vi "sortByChannel.vi"(8 "error in (no error)":errorcluster, 11 "RfOutputData in":refnum<class "RfOutputData.lvclass">) -> (0 "error out":errorcluster, 2 "sortedData":T1(array[cluster]), 3 "RfOutputData out":refnum<class "RfOutputData.lvclass">)   [LabVIEW 2009, in "DataMappers.lvlib" / "RfOutputData.lvclass"]
uses:
  RfOutputData.lvclass
  DatabaseHelpers/Database Objects/Channel/RfOutputChannel/RfOutputChannel.lvclass
  RfOutputData.lvclass/RfOutputData.ctl
  DatabaseHelpers/Database Objects/Channel/Channel.lvclass
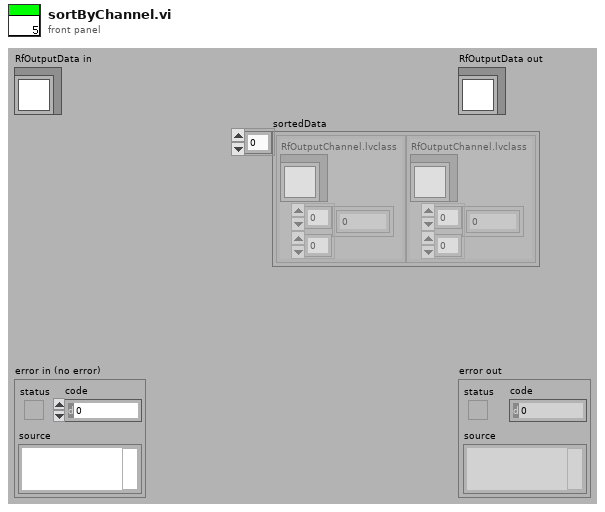
[diagram p1: front panel]
types:
  T1 = cluster{"RfOutputChannel.lvclass":refnum<class "RfOutputChannel.lvclass">, dbl[][]}[]
  T2 = cluster{"rfChannel":refnum<class "RfOutputChannel.lvclass">, "dataValue":dbl, "calibratedFreq":dbl, "calibratedPhase":dbl, "time":dbl}[]
  T3 = cluster{"rfChannel":refnum<class "RfOutputChannel.lvclass">, "dataValue":dbl, "calibratedFreq":dbl, "calibratedPhase":dbl, "time":dbl}
  T4 = cluster{"rfChannel":refnum<class "RfOutputChannel.lvclass">, dbl[][]}
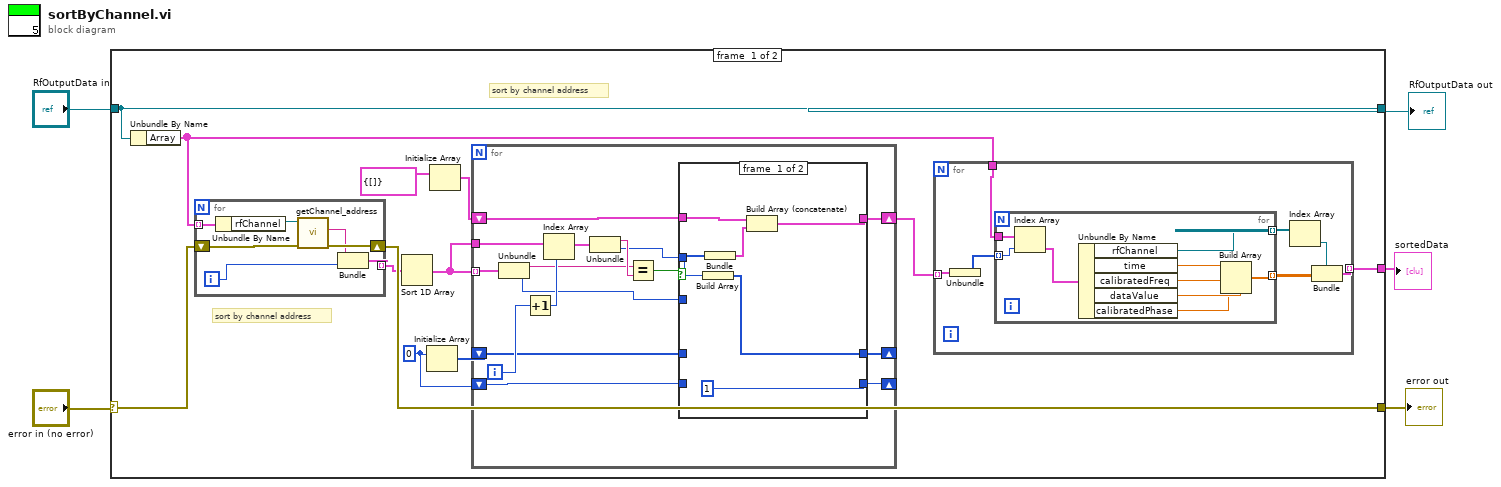
[diagram p0: block diagram]
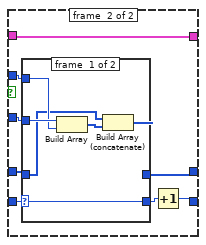
[diagram p2: hidden frame]
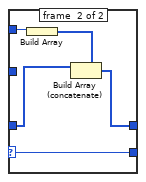
[diagram p3: hidden frame]
diagram:
  n1 = case shown="No Error" "error in (no error)" {
    selector: "error in (no error)" -> [w17 w84]
    tunnel: [w16 w84] -> w4
    tunnel: [w15 w83] -> w2
    tunnel: "RfOutputData in" -> [w15 w83]
    tunnel: [w6 _] -> w1
    frame #0 {
      w9 = 0
      # "sort by channel address"
      # "sort by channel address"
      n2 = Unbundle By Name(w15) -> ("Array"=w7:T2)
      n3 = for {
        tunnel: w7 -> [w82] mode=indexing
        shift-right: [w79] -> w16
        shift-left: w17 -> [w80]
        tunnel: [w77] -> w8 mode=indexing
        i -> [w78]
        n4 = Unbundle By Name(w82) -> ("rfChannel"=w81:refnum<class "RfOutputChannel.lvclass">)
        n5 = call "getChannel_address.vi"("error in (no error)"=w80, "Channel.lvclass in"=w81) -> ("error out"=w79:errorcluster, "channel_address"=w76:string)  [unwired: 7 in, 1 out]
        n6 = Bundle("channel_address"=w76, w78) -> (w77:cluster{"channel_address":string, i32})  [unwired: 1 in]
      }
      n7 = Sort 1D Array(array=w8) -> (sorted array=w14:cluster{"channel_address":string, i32}[])
      n8 = Initialize Array(w9) -> (w13:i32[])  [unwired: 1 in]
      n9 = Initialize Array(cluster{i32[]} {[]} ("output cluster")) -> (w11:cluster{i32[]}[])  [unwired: 1 in]
      n10 = for {
        tunnel: w14 -> [w49] mode=indexing
        tunnel: w14 -> [w48]
        shift-right: [w39] -> _
        shift-left: w9 -> [w40]
        shift-right: [w38] -> _
        shift-left: w13 -> [w37]
        shift-right: [w34] -> w10
        shift-left: w11 -> [w35]
        i -> [w47]
        n11 = Unbundle(w49) -> ("channel_address"=w36:string, w43:i32)
        n12 = Increment(x=w47) -> (x+1=w46:i32)
        n13 = Index Array(array=w48, index=w46) -> (element=w45:cluster{"channel_address":string, i32})
        n14 = Unbundle(w45) -> ("channel_address"=w42:string, w41:i32)
        n15 = Equal?(x=w36, y=w42) -> (x = y?=w44:bool)
        n16 = case shown="True" w44 {
          tunnel: w43 -> [_ w64]
          tunnel: w41 -> [w55 w63]
          tunnel: w40 -> [_ w60]
          tunnel: [1 w58] -> w39
          tunnel: [w56 w62] -> w38
          tunnel: w37 -> [w53 w61]
          tunnel: w35 -> [w52 w57]
          tunnel: [w51 w57] -> w34
          frame #0 {
            n17 = Build Array(w55) -> (w56:i32[])
            n18 = Bundle(w53) -> (w50:cluster{i32[]})  [unwired: 1 in]
            n19 = Build Array (concatenate)(w52, w50) -> (w51:cluster{i32[]}[])
          }
          frame #1 {
            n20 = case shown="0" w60 {
              selector: w60 -> [w65 w71]
              tunnel: w64 -> [w70 _]
              tunnel: w63 -> [w69 w75]
              tunnel: [w67 w73] -> w62
              tunnel: w61 -> [w66 w72]
              tunnel: [w65 w71] -> w59
              frame #0 {
                n21 = Build Array(w70, w69) -> (w68:i32[])
                n22 = Build Array (concatenate)(w66, w68) -> (w67:i32[])
              }
              frame #1 {
                n23 = Build Array(w75) -> (w74:i32[])
                n24 = Build Array (concatenate)(w72, w74) -> (w73:i32[])
              }
            }
            n25 = Increment(x=w59) -> (x+1=w58:i32)
          }
        }
      }
      n26 = for {
        tunnel: w10 -> [w24] mode=indexing
        tunnel: w7 -> [w23]
        tunnel: [w21] -> w6 mode=indexing
        n27 = Unbundle(w24) -> (w22:i32[])
        n28 = for {
          tunnel: w23 -> [w33]
          tunnel: w22 -> [w32] mode=indexing
          tunnel: [w30] -> w20 mode=indexing
          tunnel: [w25] -> w18 mode=indexing
          n29 = Index Array(array=w33, index=w32) -> (element=w31:T3)
          n30 = Unbundle By Name(w31) -> ("rfChannel"=w30:refnum<class "RfOutputChannel.lvclass">, "time"=w29:dbl, "calibratedFreq"=w28:dbl, "dataValue"=w27:dbl, "calibratedPhase"=w26:dbl)
          n31 = Build Array(w29, w28, w27, w26) -> (w25:dbl[])
        }
        n32 = Index Array(array=w20) -> (element=w19:refnum<class "RfOutputChannel.lvclass">)  [unwired: 1 in]
        n33 = Bundle("rfChannel"=w19, w18) -> (w21:T4)  [unwired: 1 in]
      }
    }
    frame #1 {
    }
  }
  "error out" <- w4
  "RfOutputData out" <- w2
  "sortedData" <- w1
